vi "FTW-ActorRef-SpawnNewActor.vi"(0 "Actor Ref Prototype":refnum<class "FTW-Actor-Bootstrapper.lvclass">, 11 "error in":errorcluster) -> (4 "Actor Reference":refnum<class "FTW-Actor-Bootstrapper.lvclass">, 15 "error out":errorcluster)   [LabVIEW 2012, in "FTW-Actor-Bootstrapper.lvclass"]
uses:
  FTW-Actor-Bootstrapper.lvclass
  Reference/FTW-ActorReference.lvclass
panel:
  # "Inputs"
  # "Outputs"
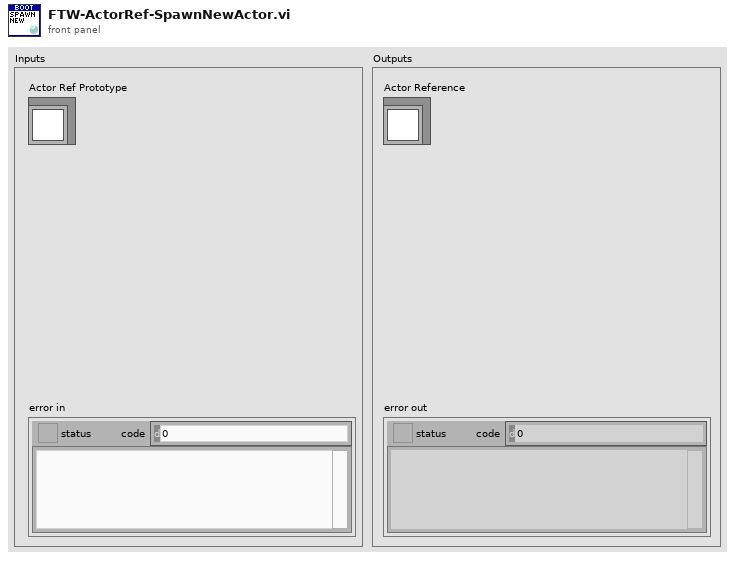
[diagram p1: front panel]
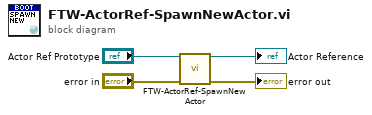
[diagram p0: block diagram]
diagram:
  n1 = call-parent "FTW-ActorRef-SpawnNewActor.vi"("Actor Ref Prototype"="Actor Ref Prototype", "error in"="error in") -> ("Actor Reference"=→"Actor Reference":refnum<class "FTW-Actor-Bootstrapper.lvclass">, "error out"=→"error out":errorcluster)  [unwired: 12 in]
